vi "Toggle.vi"(10 "Input 2":bool, 11 "Input":bool) -> (2 "Output 2":bool, 3 "Output":bool)   [LabVIEW 2018]
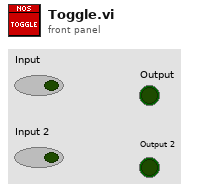
[diagram p1: front panel]
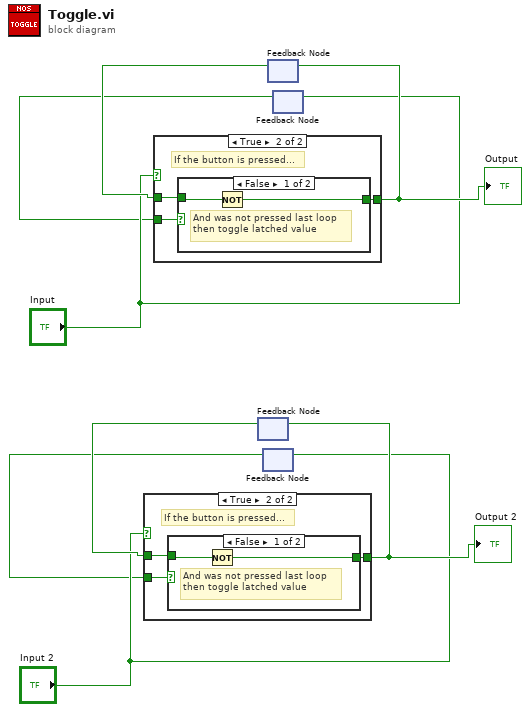
[diagram p0: block diagram]
diagram:
  n1 = feedback #1() -> (w3:bool)  [unwired: 1 in]
  n2 = feedback #2() -> (w1:bool)  [unwired: 1 in]
  n3 = case shown="True" "Input 2" {
    tunnel: w1 -> [_ w12]
    tunnel: w3 -> [w9 w11]
    tunnel: [w9 w10] -> w4
    frame False {
      # "then do nothing"
      # "If button is not pressed"
    }
    frame True {
      # "If the button is pressed..."
      n4 = case shown="False" w12 {
        tunnel: w11 -> [w13 w15]
        tunnel: [w14 w15] -> w10
        frame False {
          # "And was not pressed last loop\nthen toggle latched value"
          n5 = Not(x=w13) -> (.not. x?=w14:bool)
        }
        frame True {
          # "And was pressed last loop\nthen hold current latched value"
        }
      }
    }
  }
  "Output 2" <- w4
  n6 = feedback-in #1(w4) -> ()
  n7 = feedback-in #2("Input 2") -> ()
  n8 = feedback #3() -> (w7:bool)  [unwired: 1 in]
  n9 = feedback-in #4("Input") -> ()
  n10 = feedback #4() -> (w5:bool)  [unwired: 1 in]
  n11 = case shown="True" "Input" {
    tunnel: w5 -> [_ w19]
    tunnel: w7 -> [w16 w18]
    tunnel: [w16 w17] -> w8
    frame False {
      # "then do nothing"
      # "If button is not pressed"
    }
    frame True {
      # "If the button is pressed..."
      n12 = case shown="False" w19 {
        tunnel: w18 -> [w20 w22]
        tunnel: [w21 w22] -> w17
        frame False {
          # "And was not pressed last loop\nthen toggle latched value"
          n13 = Not(x=w20) -> (.not. x?=w21:bool)
        }
        frame True {
          # "And was pressed last loop\nthen hold current latched value"
        }
      }
    }
  }
  "Output" <- w8
  n14 = feedback-in #3(w8) -> ()
